vi "Get AutoVision Device Bitfilepath.vi"(8 "error in (no error)":errorcluster, 11 "Device Resource":string) -> (0 "error out":errorcluster, 3 "Bitfile path":path, 5 "Device found":bool)   [LabVIEW 2025, in "Automotive Vision.lvclass"]
uses:
  Automotive Vision.lvclass
  Automotive Vision.lvclass/Automotive Vision.ctl
  <vilib>/nisyscfg/nisyscfg.lvlib
  <vilib>/nisyscfg/Filter Mode.ctl
  <resource>/objmgr/niflexrioatomicsae.rc
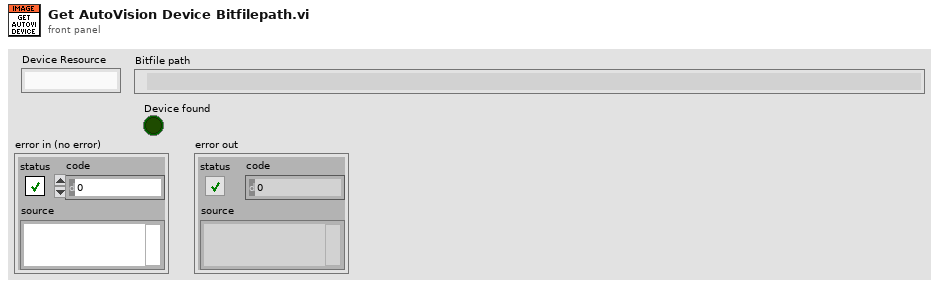
[diagram p1: front panel]
types:
  T1 = typedef "nisyscfg.lvlib/Filter Mode.ctl" = i32
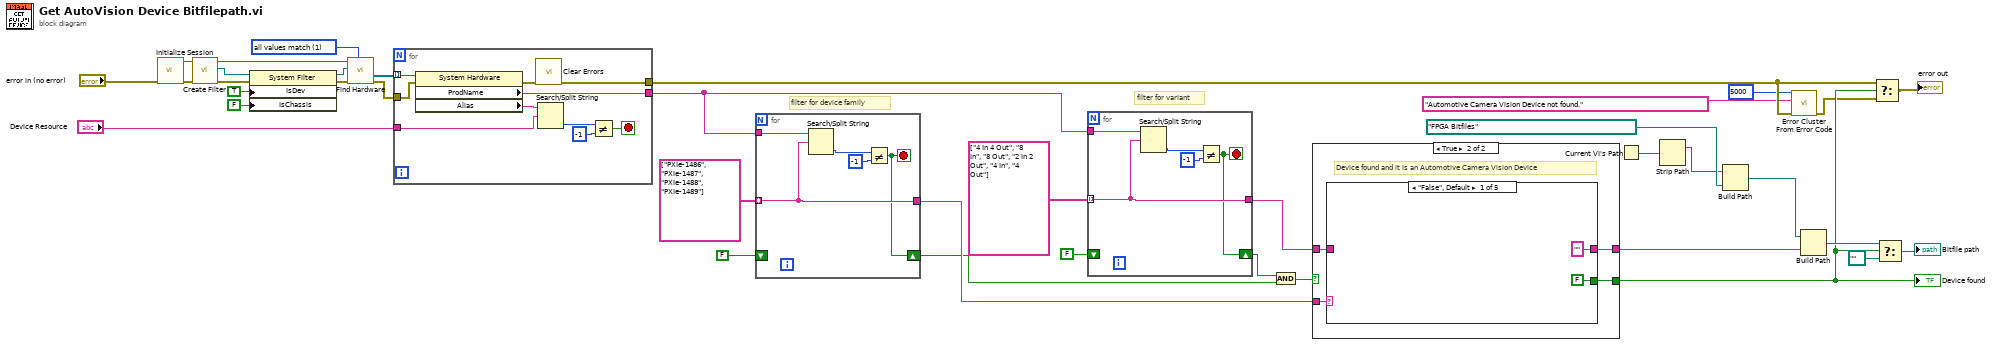
[diagram p0: block diagram]
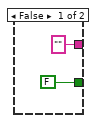
[diagram p2: hidden frame]
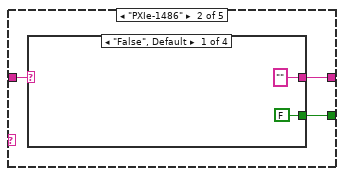
[diagram p3: hidden frame]
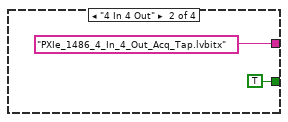
[diagram p4: hidden frame]
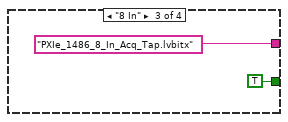
[diagram p5: hidden frame]
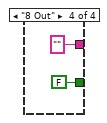
[diagram p6: hidden frame]
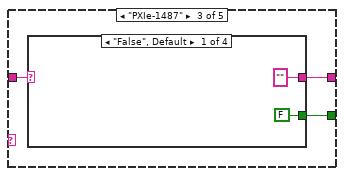
[diagram p7: hidden frame]
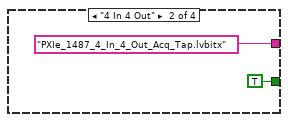
[diagram p8: hidden frame]
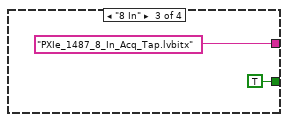
[diagram p9: hidden frame]
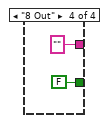
[diagram p10: hidden frame]
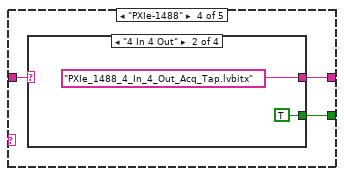
[diagram p11: hidden frame]
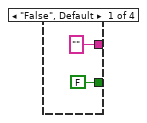
[diagram p12: hidden frame]
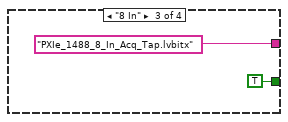
[diagram p13: hidden frame]
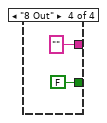
[diagram p14: hidden frame]
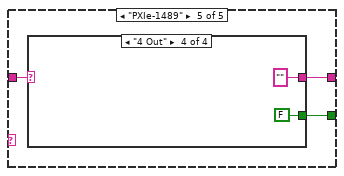
[diagram p15: hidden frame]
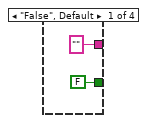
[diagram p16: hidden frame]
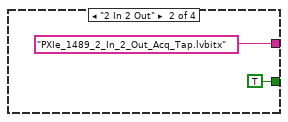
[diagram p17: hidden frame]
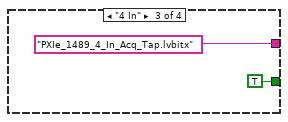
[diagram p18: hidden frame]
diagram:
  w30 = T1 1 items=["all values match"=1, "any value matches"=2, "values do not match"=3, "all properties exist"=4] ("Filter Mode (all values match)")
  # "filter for variant"
  # "filter for device family"
  n1 = call <vilib>:"Initialize Session.vi"("error in (no error)"="error in (no error)") -> ("error out"=w33:errorcluster, "Session out"=w36:refnum<k21>)  [unwired: 9 in]
  n2 = call <vilib>:"Create Filter.vi"("error in (no error)"=w33, "Session in"=w36) -> ("error out"=w31:errorcluster, "Filter out"=w32:refnum<k20>, "Session out"=w37:refnum<k21>)  [unwired: 7 in]
  n3 = property class="System Filter"(reference=w32, error in=w31, "IsDev"=TRUE ("Is Chassis"), "IsChassis"=FALSE ("Is Chassis")) -> (reference out=w27:refnum<k20>, error out=w38:errorcluster)
  n4 = call <vilib>:"Find Hardware.vi"("Filter Mode (all values match)"=w30, "error in (no error)"=w38, "Filter in"=w27, "Session in"=w37) -> ("error out"=w28:errorcluster, "Resources out"=w29:refnum<k20>[])  [unwired: 4 in, 2 out]
  n5 = for {
    tunnel: w29 -> [w47] mode=indexing
    tunnel: "Device Resource" -> [w46]
    tunnel: w28 -> [w45]
    tunnel: [w44] -> w5
    tunnel: [w39] -> w21
    stop <- w40 stop-if-true
    n6 = property class="System Hardware"(reference=w47, error in=w45) -> (error out=w48:errorcluster, "ProdName"=w39:string, "Alias"=w41:string)  [unwired: 1 out]
    n7 = call <vilib>:"Clear Errors.vi"("error in (no error)"=w48) -> ("error out"=w44:errorcluster)  [unwired: 5 in, 1 out]
    n8 = Search/Split String(string=w41, search string/char (-)=w46) -> (offset of match=w43:i32)  [unwired: 1 in, 2 out]
    n9 = Not Equal?(x=w43, y=-1) -> (x != y?=w40:bool)
  }
  n10 = for {
    tunnel: w21 -> [w53]
    tunnel: string[] ["PXIe-1486", "PXIe-1487", "PXIe-1488", "PXIe-1489"] -> [w50] mode=indexing
    tunnel: [w50] -> w20
    shift-right: [w49] -> w18
    shift-left: FALSE -> [_]
    stop <- w49 stop-if-true
    n11 = Search/Split String(string=w53, search string/char (-)=w50) -> (offset of match=w51:i32)  [unwired: 1 in, 2 out]
    n12 = Not Equal?(x=w51, y=-1) -> (x != y?=w49:bool)
  }
  n13 = for {
    tunnel: w21 -> [w58]
    tunnel: string[] ["4 In 4 Out", "8 In", "8 Out", "2 In 2 Out", "4 In", "4 Out"] -> [w55] mode=indexing
    tunnel: [w55] -> w16
    shift-right: [w54] -> w19
    shift-left: FALSE -> [_]
    stop <- w54 stop-if-true
    n14 = Search/Split String(string=w58, search string/char (-)=w55) -> (offset of match=w56:i32)  [unwired: 1 in, 2 out]
    n15 = Not Equal?(x=w56, y=-1) -> (x != y?=w54:bool)
  }
  n16 = And(x=w19, y=w18) -> (x .and. y?=w17:bool)
  n17 = case shown="True" w17 {
    tunnel: w20 -> [_ w64]
    tunnel: w16 -> [_ w63]
    tunnel: ["" w62] -> w15
    tunnel: [FALSE w61] -> w7
    frame False {
    }
    frame True {
      # "Device found and it is an Automotive Camera Vision Device"
      n18 = case shown="\"False\", Default" w64 {
        tunnel: w63 -> [_ w69 w80 w91 w102]
        tunnel: ["" w68 w79 w90 w101] -> w62
        tunnel: [FALSE w67 w78 w89 w100] -> w61
        frame "False", Default {
        }
        frame "PXIe-1486" {
          n19 = case shown="\"False\", Default" w69 {
            tunnel: ["" "PXIe_1486_4_In_4_Out_Acq_Tap.lvbitx" "PXIe_1486_8_In_Acq_Tap.lvbitx" ""] -> w68
            tunnel: [FALSE TRUE TRUE FALSE] -> w67
            frame "False", Default {
            }
            frame "4 In 4 Out" {
            }
            frame "8 In" {
            }
            frame "8 Out" {
            }
          }
        }
        frame "PXIe-1487" {
          n20 = case shown="\"False\", Default" w80 {
            tunnel: ["" "PXIe_1487_4_In_4_Out_Acq_Tap.lvbitx" "PXIe_1487_8_In_Acq_Tap.lvbitx" ""] -> w79
            tunnel: [FALSE TRUE TRUE FALSE] -> w78
            frame "False", Default {
            }
            frame "4 In 4 Out" {
            }
            frame "8 In" {
            }
            frame "8 Out" {
            }
          }
        }
        frame "PXIe-1488" {
          n21 = case shown="\"4 In 4 Out\"" w91 {
            tunnel: ["" "PXIe_1488_4_In_4_Out_Acq_Tap.lvbitx" "PXIe_1488_8_In_Acq_Tap.lvbitx" ""] -> w90
            tunnel: [FALSE TRUE TRUE FALSE] -> w89
            frame "False", Default {
            }
            frame "4 In 4 Out" {
            }
            frame "8 In" {
            }
            frame "8 Out" {
            }
          }
        }
        frame "PXIe-1489" {
          n22 = case shown="\"4 Out\"" w102 {
            tunnel: ["" "PXIe_1489_2_In_2_Out_Acq_Tap.lvbitx" "PXIe_1489_4_In_Acq_Tap.lvbitx" ""] -> w101
            tunnel: [FALSE TRUE TRUE FALSE] -> w100
            frame "False", Default {
            }
            frame "2 In 2 Out" {
            }
            frame "4 In" {
            }
            frame "4 Out" {
            }
          }
        }
      }
    }
  }
  "Device found" <- w7
  n23 = Current VI's Path() -> (path=w9:path)
  n24 = Strip Path(path=w9) -> (stripped path=w8:path)  [unwired: 1 out]
  n25 = Build Path(base path=w8, name or relative path=path "FPGA Bitfiles" ("base path")) -> (appended path=w10:path)
  n26 = call <vilib>:"Error Cluster From Error Code.vi"("error in (no error)"=w5, "error message (\"\")"="Automotive Camera Vision Device not found." ("error message (\"\")"), "error code (0)"=5000) -> ("error out"=w6:errorcluster)  [unwired: 6 in]
  n27 = Build Path(base path=w10, name or relative path=w15) -> (appended path=w14:path)
  n28 = Select(t=w5, s=w7, f=w6) -> (s? t:f=→"error out":errorcluster)
  n29 = Select(t=w14, s=w7, f=path "") -> (s? t:f=→"Bitfile path":path)
